vi "CFTS-Restore Panel.vi"(0 "State (in)":T1, 5 "VI refnum":refnum<vi>, 9 "Restore?":bool, 11 "error in (no error)":errorcluster) -> (4 "State":T1, 15 "error out":errorcluster)   [LabVIEW 2020]
uses:
  CFTS-Experiment State.ctl
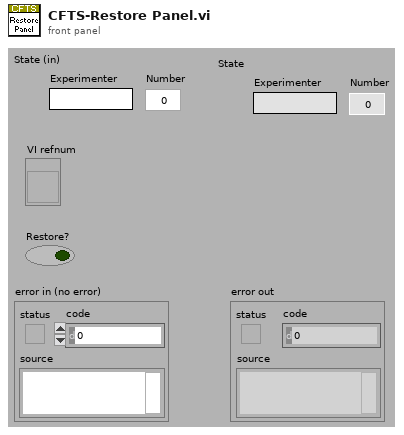
[diagram p1: front panel]
types:
  T1 = typedef "CFTS-Experiment State.ctl" = cluster{"Experimenter":string, "Number":u32, "Right":string, "Left":string, "Data Folder":path, "State File":path, "Version Info":string, "End Exposure Time":dbl, "Exposure Duration":string, "Run #":cluster{"CAP":i16, "ABR":i16, "DP":i16, "VsEP":i16, "MeasSeq":i16, "SubSeq":i16, "SFOAE":i16}}
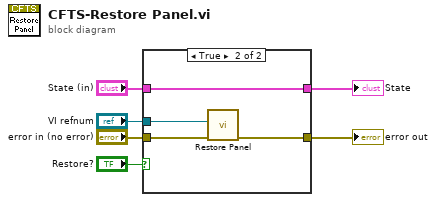
[diagram p0: block diagram]
diagram:
  n1 = case shown="True" "Restore?" {
    tunnel: "error in (no error)" -> [w7 w12]
    tunnel: "VI refnum" -> [_ w11]
    tunnel: "State (in)" -> [w8 w10]
    tunnel: [w8 w10] -> w3
    tunnel: [w7 w9] -> w2
    frame False {
    }
    frame True {
      n2 = call "Restore Panel.vi"("Error In"=w12, "VI reference"=w11) -> ("error out"=w9:errorcluster)  [unwired: 9 in]
    }
  }
  "error out" <- w2
  "State" <- w3
